vi "FM-Frequency Modulation-Sound Output.vi"() -> ()   [LabVIEW 2016]
uses:
  <vilib>/sound2/lvsound2.llb/Sound Data Format.ctl
  <vilib>/Platform/TimedLoop/XDataNode/timing_clust.ctl
  <vilib>/Platform/TimedLoop/XDataNode/nitl_modes.ctl
  <vilib>/Platform/TimedLoop/XDataNode/wakeup.ctl
  <vilib>/express/express analysis/Spectral/Block/exnSpectralBlock spectral measurements power poly.vi
  <vilib>/express/express analysis/Spectral/Block/exnSpectralBlock spectral measurements power DDT.vi
  <vilib>/sound2/lvsound2.llb/Sound Output Write (DBL Single).vi
  <vilib>/Platform/TimedLoop/XDataNode/XDataNode.xnode
  <vilib>/express/express analysis/Spectral/XNode/ExpressSpectralMeasurementsBlockNode.xnode
  <vilib>/measure/NI_MABase.lvlib
  <vilib>/Platform/TimedLoop/XDataNode/XDNodeRunTimeDep.lvlib
panel:
  in  "device ID":u32
  out "FM Wave in Frequency Domain":dynamicdata(graph)=[{"t0"=timestamp(0 s since 1904-01-01), "dt"=12.5, "Y"=array[400 elements], "attributes"=variant("NI_ChannelName"=variant(string "Power Spectrum"))}]
  out "FM Wave in Time Domain":waveform(dbl)(graph)={"t0"=timestamp(0 s since 1904-01-01), "dt"=0.0001, "Y"=array[800 elements]}
  in  "FM Deviation (Hz)":dbl(slide)=200.0 min=1.0 max=1000.0 scale=1.0..400.0 scale format="%#_6p"
  in  "Baseband Frequency (Hz)":dbl(slide)=200.0 min=50.0 max=1000.0 scale=50.0..1000.0 scale format="%#_6p"
  out "Baseband Wave (Time Domain)":waveform(dbl)(graph)={"t0"=timestamp(0 s since 1904-01-01), "dt"=0.0001, "Y"=array[800 elements]}
  out "Carrier Wave (Time Domain)":waveform(dbl)(graph)={"t0"=timestamp(0 s since 1904-01-01), "dt"=0.0001, "Y"=array[800 elements]}
  in  "Carrier Frequency (Hz)":dbl(slide)=400.0 min=50.0 max=1000.0 scale=200.0..1000.0 scale format="%#_6p"
  in  "stop":bool
  # "FM - Frequency Modulation"
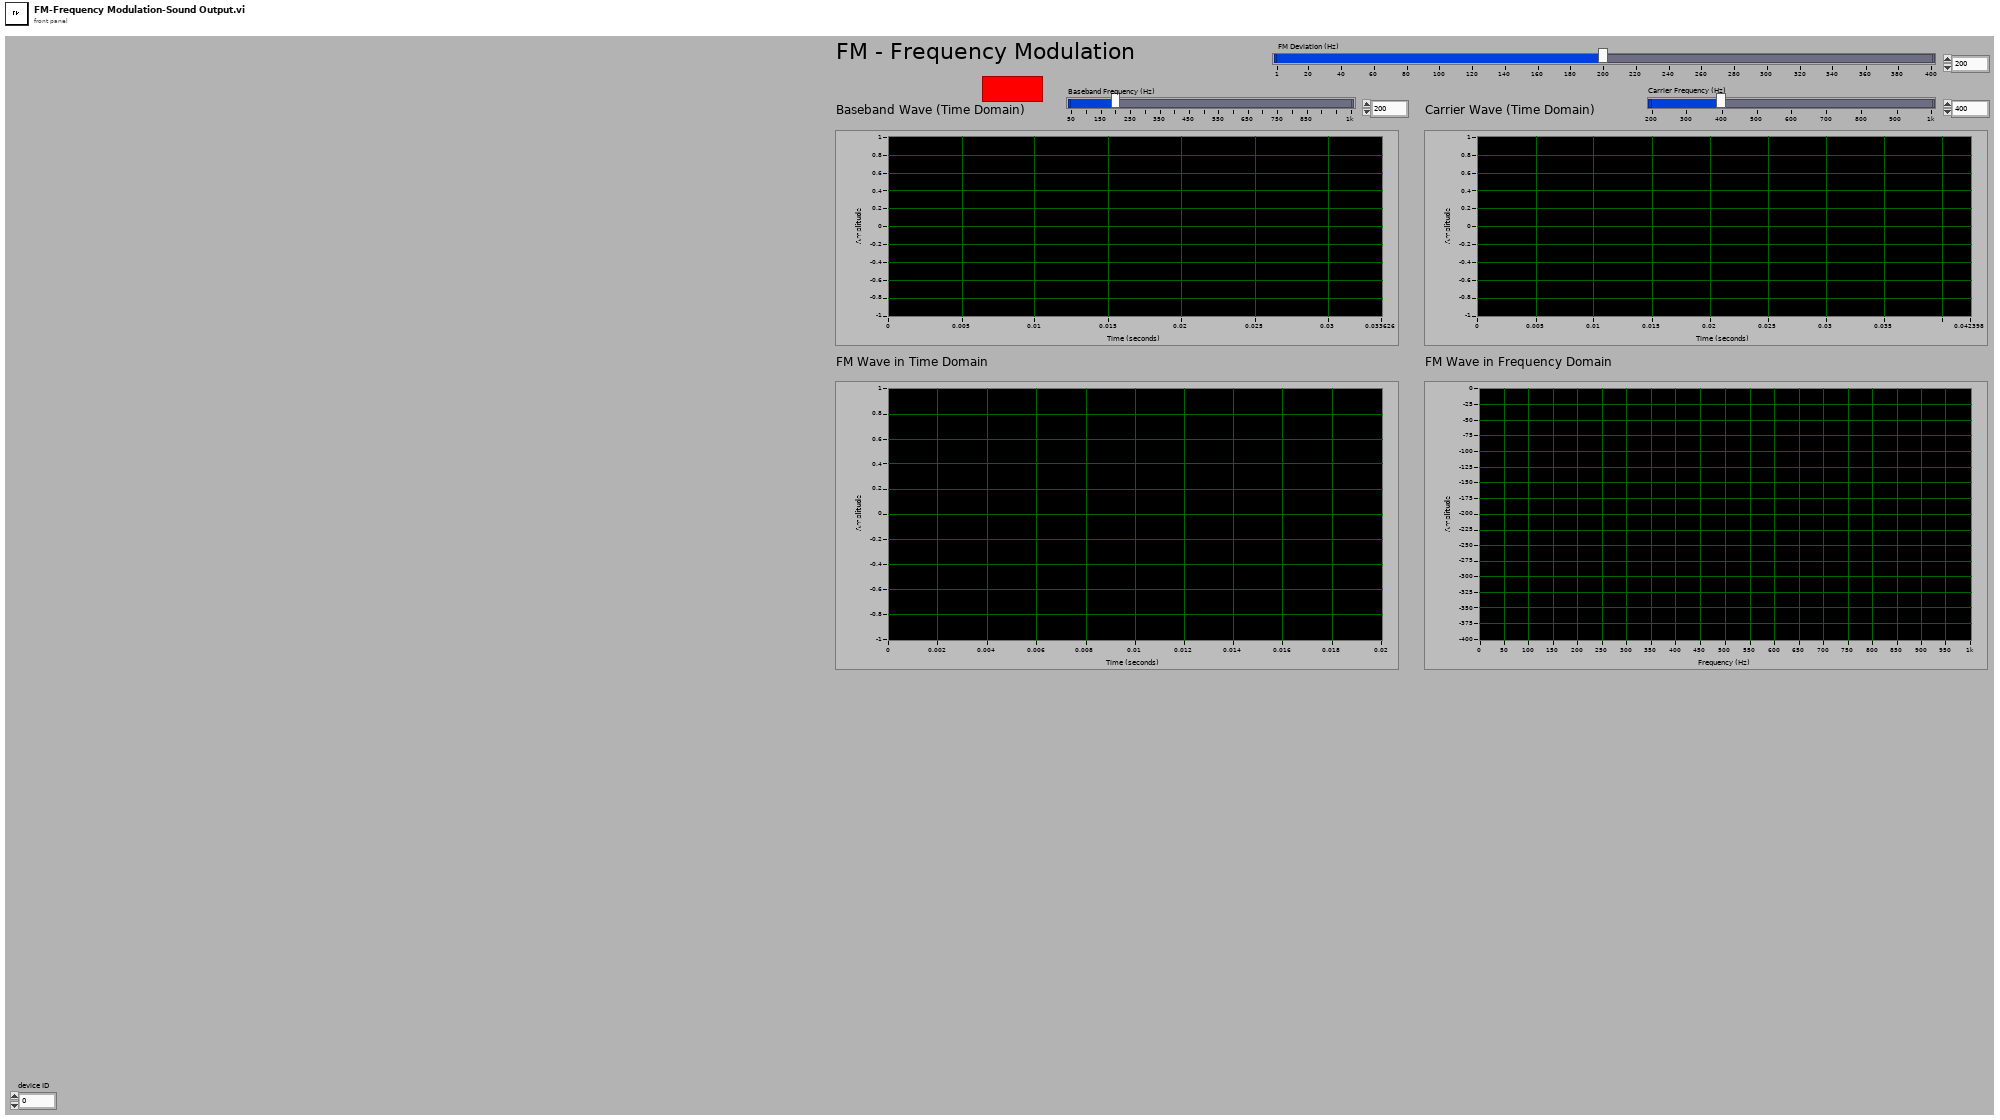
[diagram p1: front panel]
types:
  T1 = typedef "Sound Data Format.ctl" = cluster{"sample rate (S/s)":dbl, "number of channels":i32, "bits per sample":i32}
  T2 = typedef "Sound Output Task ID.ctl" = u32
  T3 = typedef "XDNodeRunTimeDep.lvlib/timing_clust.ctl" = cluster{"Expected End [f-1]":u64, "Actual End [f-1]":u64, "Finished Late? [f-1]":bool, "Expected End [i-1]":u64, "Actual End [i-1]":u64, "Finished Late? [i-1]":bool, "Expected Start [i]":u64, "Actual Start [i]":u64, "Expected Start [f]":u64, "Actual Start [f]":u64, "Source Name":string, "Structure Name":string, "Period":i64, "Deadline":i64, "Offset":i64, "Start":i64, "Priority":i32, "Timeout":i32, "Mode":T4, "Wakeup Reason":T5, "Error":errorcluster, "Source Type":string, "Secondary Source Type":string, "Global End Time":u64, "Global Start Time":u64, "Frame Duration":u64, "Iteration Duration":u64, "Assigned CPU":i32, "I/O Scan Engine Mode":u32}
  T4 = typedef "XDNodeRunTimeDep.lvlib/nitl_modes.ctl" = enum32{"No Change", "Process missed periods, maintain original phase", "Discard missed periods, maintain original phase", "Process missed periods, ignore original phase", "Discard missed periods, ignore original phase"}
  T5 = typedef "XDNodeRunTimeDep.lvlib/wakeup.ctl" = enum32{"Normal", "Aborted", "Asynchronous wakeup", "Timing source error", "Timed loop error", "Timeout"}
  T6 = cluster{"averaging mode":u16, "weighting mode":u16, "number of averages":u32}
  T7 = cluster{"dB On (F)":bool, "unwrap phase (F)":bool, "convert to degree (F)":bool}
  T8 = cluster{"sample rate (S/s)":dbl, "sample rate (S/s)":dbl}
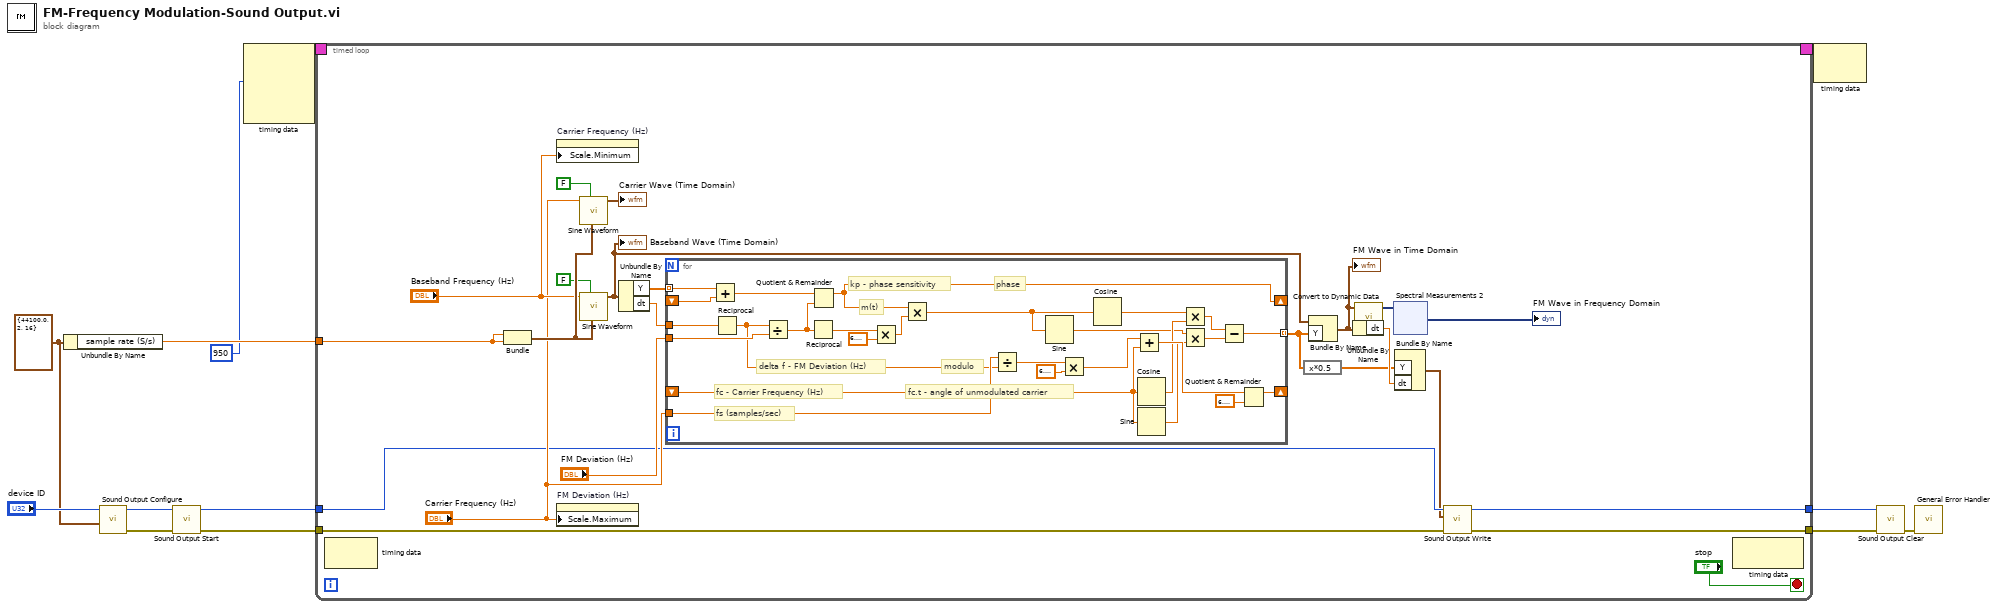
[diagram p0: block diagram]
diagram:
  w10 = T1 {"sample rate (S/s)"=44100.0, "number of channels"=2, "bits per sample"=16} ("sound format")
  n1 = Unbundle By Name(w10) -> ("sample rate (S/s)"=w7:dbl)
  n2 = call <vilib>:"Sound Output Configure.vi"("sound format"=w10, "device ID"="device ID") -> ("error out"=w11:errorcluster, "task ID"=w12:T2)  [unwired: 8 in]
  n3 = call <vilib>:"Sound Output Start.vi"("error in (no error)"=w11, "task ID"=w12) -> ("error out"=w9:errorcluster, "task ID out"=w8:T2)  [unwired: 8 in]
  n4 = node-c288(i64 950 ("Period")) -> (w3:T3)  [unwired: 3 in]
  n5 = timed-loop {
    tunnel: [w19] -> w6
    tunnel: [w20] -> w5
    tunnel: w8 -> [w22]
    tunnel: w9 -> [w21]
    tunnel: w7 -> [w23]
    timing: w3 -> [_]
    timing-out: [_] -> w2
    stop <- "stop" stop-if-true
    n6 = node-c288() -> ()  [unwired: 1 in, 1 out]
    n7 = Bundle("sample rate (S/s)"=w23, "sample rate (S/s)"=w23) -> (w32:T8)  [unwired: 1 in]
    n8 = property on="Carrier Frequency (Hz)" class="Slide (strict)"("Scale.Minimum"="Baseband Frequency (Hz)") -> ()  [unwired: 2 in, 2 out]
    n9 = property on="FM Deviation (Hz)" class="Slide (strict)"("Scale.Maximum"="Carrier Frequency (Hz)") -> ()  [unwired: 2 in, 2 out]
    n10 = call <vilib>:"Sine Waveform.vi"("sampling info"=w32, "reset signal"=FALSE, "frequency"="Carrier Frequency (Hz)") -> ("signal out"=→"Carrier Wave (Time Domain)":waveform(dbl))  [unwired: 7 in, 1 out]
    n11 = call <vilib>:"Sine Waveform.vi"("sampling info"=w32, "reset signal"=FALSE, "frequency"="Baseband Frequency (Hz)") -> ("signal out"=w33:waveform(dbl))  [unwired: 7 in, 1 out]
    "Baseband Wave (Time Domain)" <- w33
    n12 = Unbundle By Name(w33) -> ("Y"=w36:dbl[], "dt"=w34:dbl)
    n13 = for {
      tunnel: w34 -> [w74]
      tunnel: "FM Deviation (Hz)" -> [w73]
      shift-right: [w58] -> _
      shift-left: _ -> [w57]
      tunnel: w36 -> [w56] mode=indexing
      tunnel: "Carrier Frequency (Hz)" -> [w70]
      tunnel: [w65] -> w15 mode=indexing
      shift-right: [w61] -> _
      shift-left: _ -> [w54]
      # "fc.t - angle of unmodulated carrier"
      # "m(t)"
      # "fc - Carrier Frequency (Hz)"
      # "delta f - FM Deviation (Hz)"
      # "phase"
      # "kp - phase sensitivity"
      # "modulo"
      # "fs (samples/sec)"
      n14 = Add(x=w56, y=w57) -> (x+y=w60:dbl)
      n15 = Reciprocal(x=w74) -> (1/x=w69:dbl)
      n16 = Divide(x=w69, y=w73) -> (x/y=w59:dbl)
      n17 = Reciprocal(x=w59) -> (1/x=w48:dbl)
      n18 = Quotient & Remainder(x=w60, y=w59) -> (x-y*floor(x/y)=w58:dbl)  [unwired: 1 out]
      n19 = Multiply(x=w48, y=6.283185307179586) -> (x*y=w71:dbl)
      n20 = Multiply(x=w58, y=w71) -> (x*y=w49:dbl)
      n21 = Divide(x=w70, y=w69) -> (x/y=w67:dbl)
      n22 = Sine(x=w49) -> (sin(x)=w50:dbl)
      n23 = Multiply(x=w67, y=6.283185307179586) -> (x*y=w64:dbl)
      n24 = Cosine(x=w49) -> (cos(x)=w52:dbl)
      n25 = Add(x=w64, y=w54) -> (x+y=w63:dbl)
      n26 = Cosine(x=w54) -> (cos(x)=w51:dbl)
      n27 = Sine(x=w54) -> (sin(x)=w53:dbl)
      n28 = Multiply(x=w52, y=w51) -> (x*y=w66:dbl)
      n29 = Multiply(x=w50, y=w53) -> (x*y=w55:dbl)
      n30 = Subtract(x=w66, y=w55) -> (x-y=w65:dbl)
      n31 = Quotient & Remainder(x=w63, y=6.283185307179586) -> (x-y*floor(x/y)=w61:dbl)  [unwired: 1 out]
    }
    n32 = expression code="x*0.5"(w15) -> (w14:dbl[])
    n33 = Bundle By Name(cluster=w33, "Y"=w15) -> (w17:waveform(dbl))
    "FM Wave in Time Domain" <- w17
    n34 = Unbundle By Name(w17) -> ("dt"=w16:dbl)
    n35 = call "Convert to Dynamic Data"("Waveform"=w17) -> ("Dynamic Data Type"=w24:dynamicdata)  [unwired: 3 in]
    n36 = xnode "Spectral Measurements 2"("Signals"=w24) -> ("Power Spectrum"=→"FM Wave in Frequency Domain":dynamicdata)  [unwired: 1 in, 1 out]
    n37 = Bundle By Name("Y"=w14, "dt"=w16) -> (w18:waveform(dbl))  [unwired: 1 in]
    n38 = call-poly <vilib>:"Sound Output Write.vi"("error in (no error)"=w21, "data"=w18, "task ID"=w22) -> ("error out"=w20:errorcluster, "task ID out"=w19:T2)  [unwired: 7 in]
    n39 = node-c288() -> ()  [unwired: 1 in, 1 out]
  }
  n40 = node-c288(w2) -> ()  [unwired: 1 out]
  n41 = call <vilib>:"Sound Output Clear.vi"("error in (no error)"=w5, "task ID"=w6) -> ("error out"=w4:errorcluster)  [unwired: 9 in]
  n42 = call <vilib>:"General Error Handler.vi"("error in (no error)"=w4) -> ()  [unwired: 2 in, 13 out]
